vi "Insert Color Transform Matrix.vi"(8 "error in (no error)":errorcluster, 9 "colorTransformMatrix":sgl[](array[numeric]), 10 "index":i32, 11 "ColorProcessor reference in":refnum<k24>) -> (0 "error out":errorcluster, 3 "ColorProcessor reference out":refnum<k24>)   [LabVIEW 2015]
uses:
  C:/code/Host/Installer/Scientific Camera Interfaces/LabVIEW/64_bit/Library_X64/Thorlabs.TSI.ColorInterfaces.dll
  64_bit/Library_X64/Thorlabs.TSI.ColorInterfaces.dll
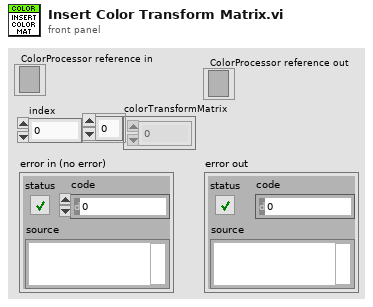
[diagram p1: front panel]
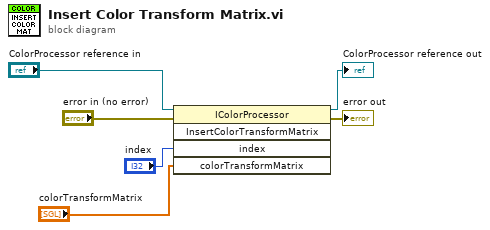
[diagram p0: block diagram]
diagram:
  n1 = invoke class="IColorProcessor" method="InsertColorTransformMatrix"(reference="ColorProcessor reference in", error in="error in (no error)", "index"="index", "colorTransformMatrix"="colorTransformMatrix") -> (reference out=→"ColorProcessor reference out":refnum<k24>, error out=→"error out":errorcluster)  [unwired: 1 in, 3 out]
